vi "measure_string.vi"() -> ()   [LabVIEW 2009]
uses:
  <instrlib>/Agilent 8000 Series/Agilent 8000 Series.lvlib
panel:
  out "std_deviation":dbl
  out "mean":dbl
  in  "Second channel":bool
  in  "Measurement Function (0: Rise Time) 2":i32(ring) caption="Measurement Function (0: Rise Time)" items=["Rise Time", "Fall Time", "Frequency", "Period", "Voltage RMS(AC)", "Voltage RMS(DC)", "Voltage RMS (AC,cycle)", "Voltage RMS (DC,cycle)", "Voltage Max", "Voltage Min", "Voltage Middle", "Voltage Vpp", "Voltage High", "Voltage Low", "Voltage Average", "Voltage Average (cycle)", "Width Negative", "Width Positive", "Duty Cycle Positive", "Amplitude", "Overshoot", "Preshoot", "Voltage Base", "Voltage Upper", "Time Max", "Time Min", "Color Grade Crossing", "Color Grade Eye Width", "Color Grade Eye Height", "Color Grade Eye Q-Factory", "Color Grade Eye Duty Cycle Distortion(Percent)", "Color Grade Eye Duty Cycle Distortion(Time)", "Color Grade Eye Jitter(PP)", "Color Grade Eye Width(RMS)", "Cycle-cycle Duty Jitter(Rising)", "Cycle-cycle Duty Jitter(Falling)", "Cycle-cycle Jitter(Rising)", "Cycle-cycle Jitter(Falling)", "Cycle-cycle - Width", "Cycle-cycle + Width", "Date Rate", "Unit Interval", "FFT Delta Frequency", "FFT Delta Magnitude", "FFT Frequency", "FFT Magnitude", "Slew Rate", "Area (Entire Display)", "Area(Single Cycle)", "Duty Cycle (Rising)", "Duty Cycle (Falling)"]
  in  "Channel (1: Channel 1) 2":i32(ring)=1 items=["Channel 1"=1, "Channel 2"=2, "Channel 3"=3, "Channel 4"=4, "Function 1"=5, "Function 2"=6, "Function 3"=7, "Function 4"=8, "Memory 1"=9, "Memory 2"=10, "Memory 3"=11, "Memory 4"=12]
  out "x-y 3":u32
  out "x-y 2":u32
  out "Numeric":i32
  out "x-y":u32
  out "output 8":dbl
  out "output 1":string
  out "remaining string":string
  out "read buffer 3":string
  out "read buffer 2":string
  out "Error Message":string
  out "Error Code":i32[](array[numeric])
  out "String":string
  in  "error in (no error)":errorcluster
  out "error out (no error)":errorcluster
  in  "VISA resource name":refnum<visa-resource-name>
  in  "Measurement Function (0: Rise Time)":i32(ring) items=["Rise Time", "Fall Time", "Frequency", "Period", "Voltage RMS(AC)", "Voltage RMS(DC)", "Voltage RMS (AC,cycle)", "Voltage RMS (DC,cycle)", "Voltage Max", "Voltage Min", "Voltage Middle", "Voltage Vpp", "Voltage High", "Voltage Low", "Voltage Average", "Voltage Average (cycle)", "Width Negative", "Width Positive", "Duty Cycle Positive", "Amplitude", "Overshoot", "Preshoot", "Voltage Base", "Voltage Upper", "Time Max", "Time Min", "Color Grade Crossing", "Color Grade Eye Width", "Color Grade Eye Height", "Color Grade Eye Q-Factory", "Color Grade Eye Duty Cycle Distortion(Percent)", "Color Grade Eye Duty Cycle Distortion(Time)", "Color Grade Eye Jitter(PP)", "Color Grade Eye Width(RMS)", "Cycle-cycle Duty Jitter(Rising)", "Cycle-cycle Duty Jitter(Falling)", "Cycle-cycle Jitter(Rising)", "Cycle-cycle Jitter(Falling)", "Cycle-cycle - Width", "Cycle-cycle + Width", "Date Rate", "Unit Interval", "FFT Delta Frequency", "FFT Delta Magnitude", "FFT Frequency", "FFT Magnitude", "Slew Rate", "Area (Entire Display)", "Area(Single Cycle)", "Duty Cycle (Rising)", "Duty Cycle (Falling)"]
  in  "Channel (1: Channel 1)":i32(ring)=1 items=["Channel 1"=1, "Channel 2"=2, "Channel 3"=3, "Channel 4"=4, "Function 1"=5, "Function 2"=6, "Function 3"=7, "Function 4"=8, "Memory 1"=9, "Memory 2"=10, "Memory 3"=11, "Memory 4"=12]
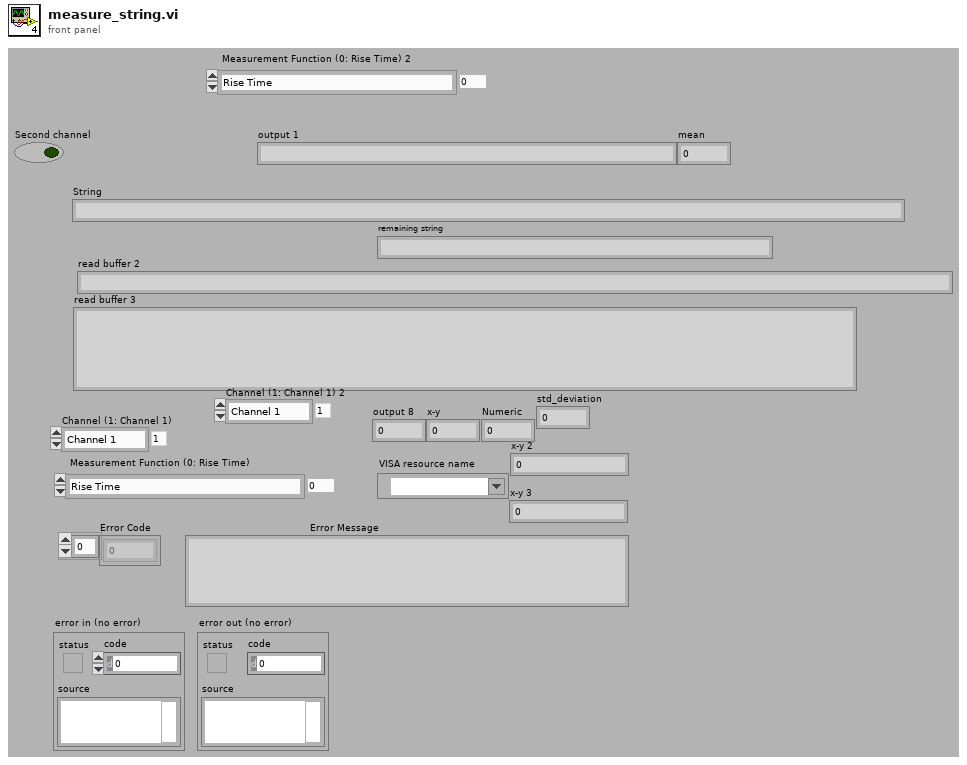
[diagram p1: front panel]
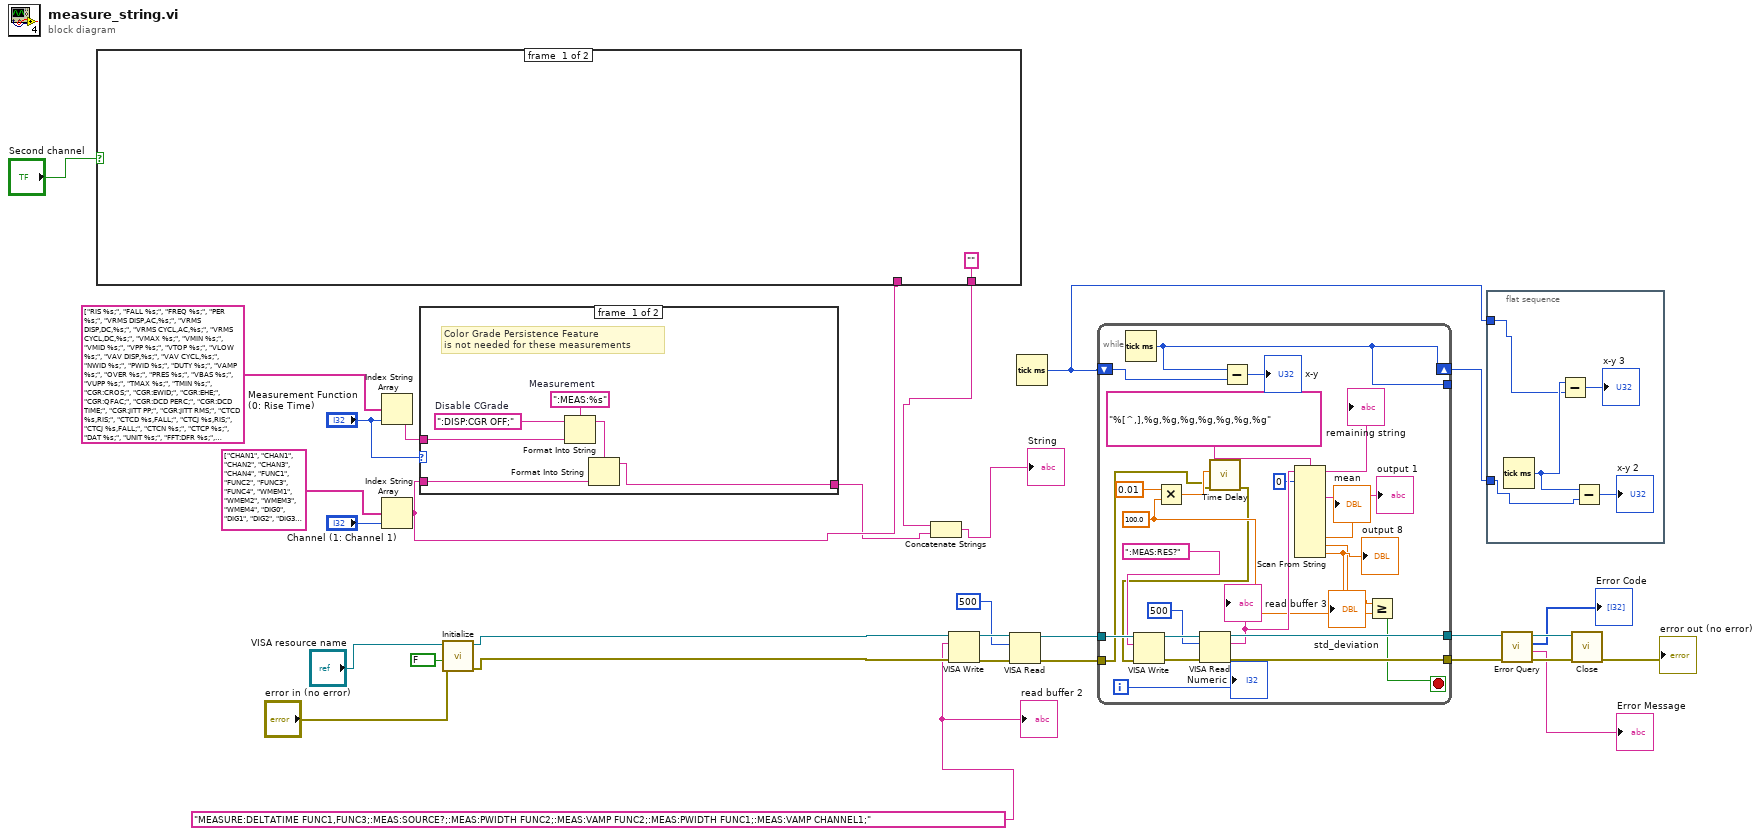
[diagram p0: block diagram]
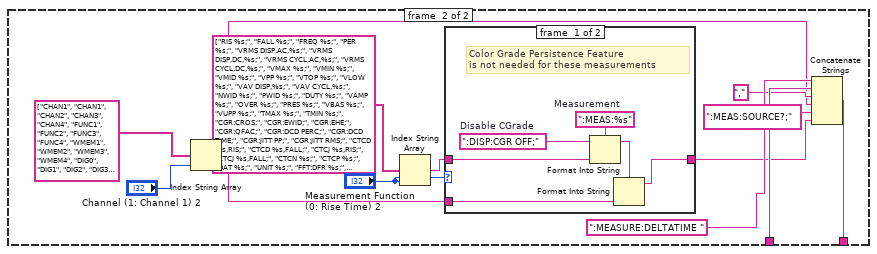
[diagram p2: hidden frame]
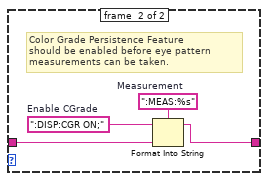
[diagram p3: hidden frame]
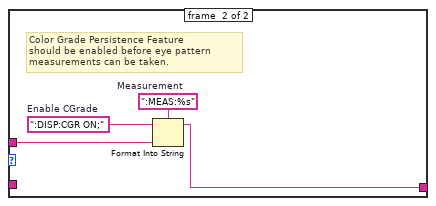
[diagram p4: hidden frame]
diagram:
  w1 = "MEASURE:DELTATIME FUNC1,FUNC3;:MEAS:SOURCE?;:MEAS:PWIDTH FUNC2;:MEAS:VAMP FUNC2;:MEAS:PWIDTH FUNC1;:MEAS:VAMP CHANNEL1;" ("write buffer")
  n1 = Index String Array(1:"Measurement Function (0: Rise Time)", 2:string[] ["RIS %s;", "FALL %s;", "FREQ %s;", "PER %s;", "VRMS DISP,AC,%s;", "VRMS DISP,DC,%s;", "VRMS CYCL,AC,%s;", "VRMS CYCL,DC,%s;", "VMAX %s;", "VMIN %s;", "VMID %s;", "VPP %s;", "VTOP %s;", "VLOW %s;", "VAV DISP,%s;", "VAV CYCL,%s;", "NWID %s;", "PWID %s;", "DUTY %s;", "VAMP %s;", "OVER %s;", "PRES %s;", "VBAS %s;", "VUPP %s;", "TMAX %s;", "TMIN %s;", "CGR:CROS;", "CGR:EWID;", "CGR:EHE;", "CGR:QFAC;", "CGR:DCD PERC;", "CGR:DCD TIME;", "CGR:JITT PP;", "CGR:JITT RMS;", "CTCD %s,RIS;", "CTCD %s,FALL;", "CTCJ %s,RIS;", "CTCJ %s,FALL;", "CTCN %s;", "CTCP %s;", "DAT %s;", "UNIT %s;", "FFT:DFR %s;", "FFT:DMAG %s;", "FFT:FREQ %s;", "FFT:MAGN %s;", "SLEW %s;", "AREA DISP,%s;", "AREA CYCL,%s;", "DUTY %s,RIS;", "DUTY %s,FALL;"]) -> (0:w30:string)  [unwired: 1 in]
  n2 = Index String Array(1:"Channel (1: Channel 1)", 2:string[] ["CHAN1", "CHAN1", "CHAN2", "CHAN3", "CHAN4", "FUNC1", "FUNC2", "FUNC3", "FUNC4", "WMEM1", "WMEM2", "WMEM3", "WMEM4", "DIG0", "DIG1", "DIG2", "DIG3", "DIG4", "DIG5", "DIG6", "DIG7", "DIG8", "DIG9", "DIG10", "DIG11", "DIG12", "DIG13", "DIG14", "DIG15", "AUX", "LINE"]) -> (0:w5:string)  [unwired: 1 in]
  n3 = case shown="True" "Second channel" {
    tunnel: ["" w38] -> w3
    tunnel: w5 -> [_ w36]
    frame #0 {
    }
    frame #1 {
      n4 = Index String Array(1:"Channel (1: Channel 1) 2", 2:string[] ["CHAN1", "CHAN1", "CHAN2", "CHAN3", "CHAN4", "FUNC1", "FUNC2", "FUNC3", "FUNC4", "WMEM1", "WMEM2", "WMEM3", "WMEM4", "DIG0", "DIG1", "DIG2", "DIG3", "DIG4", "DIG5", "DIG6", "DIG7", "DIG8", "DIG9", "DIG10", "DIG11", "DIG12", "DIG13", "DIG14", "DIG15", "AUX", "LINE"]) -> (0:w34:string)  [unwired: 1 in]
      n5 = Index String Array(1:"Measurement Function (0: Rise Time) 2", 2:string[] ["RIS %s;", "FALL %s;", "FREQ %s;", "PER %s;", "VRMS DISP,AC,%s;", "VRMS DISP,DC,%s;", "VRMS CYCL,AC,%s;", "VRMS CYCL,DC,%s;", "VMAX %s;", "VMIN %s;", "VMID %s;", "VPP %s;", "VTOP %s;", "VLOW %s;", "VAV DISP,%s;", "VAV CYCL,%s;", "NWID %s;", "PWID %s;", "DUTY %s;", "VAMP %s;", "OVER %s;", "PRES %s;", "VBAS %s;", "VUPP %s;", "TMAX %s;", "TMIN %s;", "CGR:CROS;", "CGR:EWID;", "CGR:EHE;", "CGR:QFAC;", "CGR:DCD PERC;", "CGR:DCD TIME;", "CGR:JITT PP;", "CGR:JITT RMS;", "CTCD %s,RIS;", "CTCD %s,FALL;", "CTCJ %s,RIS;", "CTCJ %s,FALL;", "CTCN %s;", "CTCP %s;", "DAT %s;", "UNIT %s;", "FFT:DFR %s;", "FFT:DMAG %s;", "FFT:FREQ %s;", "FFT:MAGN %s;", "SLEW %s;", "AREA DISP,%s;", "AREA CYCL,%s;", "DUTY %s,RIS;", "DUTY %s,FALL;"]) -> (0:w39:string)  [unwired: 1 in]
      n6 = case shown="0, Default" "Measurement Function (0: Rise Time) 2" {
        tunnel: w39 -> [w47 w52]
        tunnel: w34 -> [w45 _]
        tunnel: [w44 w50] -> w32
        frame #0 {
          w49 = ":DISP:CGR OFF;"  # Disable CGrade
          w48 = ":MEAS:%s"  # Measurement
          # "Color Grade Persistence Feature\nis not needed for these measurements"
          n7 = Format Into String(format string=w48, initial string=w49, w47) -> (resulting string=w46:string)  [unwired: 1 in, 1 out]
          n8 = Format Into String(format string=w46, w45) -> (resulting string=w44:string)  [unwired: 2 in, 1 out]
        }
        frame #1 {
          w51 = ":DISP:CGR ON;"  # Enable CGrade
          w53 = ":MEAS:%s"  # Measurement
          # "Color Grade Persistence Feature\nshould be enabled before eye pattern\nmeasurements can be taken."
          n9 = Format Into String(format string=w53, initial string=w51, w52) -> (resulting string=w50:string)  [unwired: 1 in, 1 out]
        }
      }
      n10 = Concatenate Strings(":MEASURE:DELTATIME " ("string"), w36, "," ("string"), w34, ":MEAS:SOURCE?;" ("string"), w32) -> (w38:string)
    }
  }
  n11 = case shown="27..34" "Measurement Function (0: Rise Time)" {
    tunnel: w30 -> [w57 w62]
    tunnel: w5 -> [w55 _]
    tunnel: [w54 w60] -> w2
    frame #0 {
      w59 = ":DISP:CGR OFF;"  # Disable CGrade
      w58 = ":MEAS:%s"  # Measurement
      # "Color Grade Persistence Feature\nis not needed for these measurements"
      n12 = Format Into String(format string=w58, initial string=w59, w57) -> (resulting string=w56:string)  [unwired: 1 in, 1 out]
      n13 = Format Into String(format string=w56, w55) -> (resulting string=w54:string)  [unwired: 2 in, 1 out]
    }
    frame #1 {
      w61 = ":DISP:CGR ON;"  # Enable CGrade
      w63 = ":MEAS:%s"  # Measurement
      # "Color Grade Persistence Feature\nshould be enabled before eye pattern\nmeasurements can be taken."
      n14 = Format Into String(format string=w63, initial string=w61, w62) -> (resulting string=w60:string)  [unwired: 1 in, 1 out]
    }
  }
  n15 = call <instrlib>:"Initialize.vi"("error in (no error)"="error in (no error)", "Reset (True)"=FALSE, "VISA resource name"="VISA resource name") -> ("error out"=w8:errorcluster, "VISA resource name out"=w7:refnum<visa-resource-name>)  [unwired: 7 in]
  n16 = Concatenate Strings(w3, w2) -> (→"String":string)
  n17 = VISA Write(VISA resource name=w7, write buffer=w1, error in (no error)=w8) -> (VISA resource name out=w17:refnum<visa-resource-name>, error out=w16:errorcluster)  [unwired: 1 out]
  n18 = VISA Read(VISA resource name=w17, byte count=u32 500, error in (no error)=w16) -> (VISA resource name out=w14:refnum<visa-resource-name>, error out=w13:errorcluster)  [unwired: 2 out]
  n19 = Tick Count (ms)() -> (millisecond timer value=w9:u32)
  n20 = while {
    tunnel: w14 -> [w85]
    tunnel: w13 -> [w68]
    tunnel: [w84] -> w12
    tunnel: [w83] -> w11
    tunnel: [w66] -> _
    shift-right: [w66] -> w10
    shift-left: w9 -> [w74]
    i -> [w72]
    stop <- w75 stop-if-true
    w71 = 100.0 ("y")
    n21 = Tick Count (ms)() -> (millisecond timer value=w66:u32)
    n22 = Multiply(x=0.01, y=w71) -> (x*y=w69:dbl)
    n23 = call "Time Delay"("error in (no error)"=w68, "Delay Time (s)"=w69) -> ("error out"=w67:errorcluster)  [unwired: 9 in]
    n24 = VISA Write(VISA resource name=w85, write buffer=":MEAS:RES?", error in (no error)=w67) -> (VISA resource name out=w88:refnum<visa-resource-name>, error out=w87:errorcluster)  [unwired: 1 out]
    n25 = VISA Read(VISA resource name=w88, byte count=u32 500, error in (no error)=w87) -> (VISA resource name out=w84:refnum<visa-resource-name>, read buffer=w80:string, error out=w83:errorcluster)  [unwired: 1 out]
    "read buffer 3" <- w80
    n26 = Subtract(x=w66, y=w74) -> (x-y=→"x-y":u32)
    n27 = Scan From String(format string="%[^,],%g,%g,%g,%g,%g,%g,%g", input string=w80, initial scan location=u32 0) -> (remaining string=→"remaining string":string, output 1=→"output 1":string, output 6=→"mean":dbl, output 7=→"std_deviation":dbl, output 8=w76:dbl)  [unwired: 13 in, 2 out]
    "output 8" <- w76
    n28 = Greater Or Equal?(x=w76, y=w71) -> (x >= y?=w75:bool)
    "Numeric" <- w72
  }
  n29 = flat-sequence {
    tunnel: w10 -> [w92]
    tunnel: w9 -> [w89]
    frame #0 {
      n30 = Tick Count (ms)() -> (millisecond timer value=w90:u32)
      n31 = Subtract(x=w90, y=w89) -> (x-y=→"x-y 3":u32)
      n32 = Subtract(x=w90, y=w92) -> (x-y=→"x-y 2":u32)
    }
  }
  n33 = call <instrlib>:"Error Query.vi"("error in (no error)"=w11, "VISA resource name"=w12) -> ("error out"=w24:errorcluster, "Error Message"=→"Error Message":string, "Error Code"=→"Error Code":i32[], "VISA resource name out"=w25:refnum<visa-resource-name>)  [unwired: 6 in]
  n34 = call <instrlib>:"Close.vi"("error in (no error)"=w24, "VISA resource name"=w25) -> ("error out"=→"error out (no error)":errorcluster)  [unwired: 9 in]
  "read buffer 2" <- w1
